vi "LJ Clock.vi"(10 "Sync to second":bool, 11 "Initialize":bool) -> (3 "Seconds since 1/1/1904 universal time":ext format="%.3f")   [LabVIEW 2021]
panel:
  in  "Previous Tick":u32
  in  "Seconds Offset":ext format="%.3f"
  # "Uses the combined values of \"Get Date/Time In Seconds\" and\n\"Tick Count (ms)\" to determine the absolute time (with milliseconds)\nsince midnight on January 1, 1904.\n\nSet \"Initialize\" to TRUE the first time this VI is called.\n\nsupport@labjack.com\nwww.labjack.com"
  # "If the current tick is less\nthan the previous tick, the\nmillisecond timer has rolled."
  # "Offset that must be\nadded to the millisecond\ntimer to get absolute time."
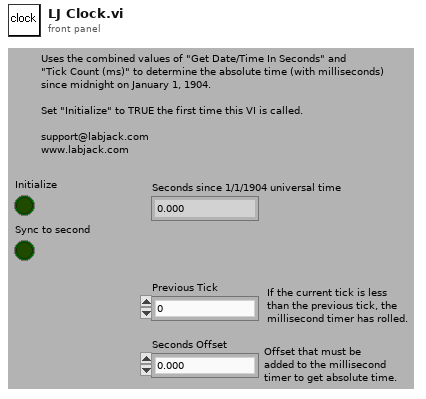
[diagram p1: front panel]
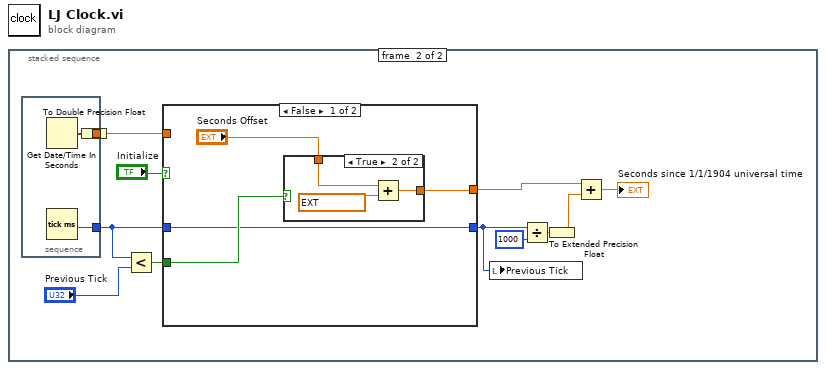
[diagram p0: block diagram]
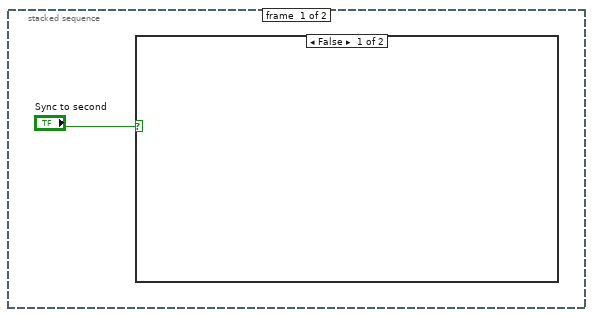
[diagram p2: hidden frame]
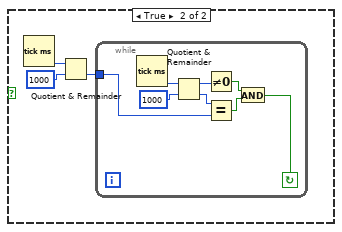
[diagram p3: hidden frame]
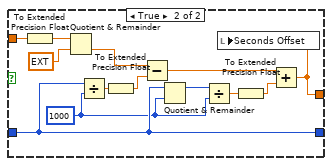
[diagram p5: hidden frame]
diagram:
  n1 = stacked-sequence {
    frame #0 {
      n2 = case shown="False" "Sync to second" {
        frame False {
        }
        frame True {
          n3 = Tick Count (ms)() -> (millisecond timer value=w3:u32)
          n4 = Quotient & Remainder(x=w3, y=u32 1000) -> (floor(x/y)=w2:u32)  [unwired: 1 out]
          n5 = while {
            tunnel: w2 -> [w8]
            stop <- w5 continue-if-true
            n6 = Tick Count (ms)() -> (millisecond timer value=w12:u32)
            n7 = Quotient & Remainder(x=w12, y=u32 1000) -> (x-y*floor(x/y)=w10:u32, floor(x/y)=w9:u32)
            n8 = Not Equal To 0?(x=w10) -> (x != 0?=w7:bool)
            n9 = Equal?(x=w9, y=w8) -> (x = y?=w6:bool)
            n10 = And(x=w7, y=w6) -> (x .and. y?=w5:bool)
          }
        }
      }
    }
    frame #1 {
      n11 = stacked-sequence {
        tunnel: [w26] -> w21
        tunnel: [w25] -> w15
        frame #0 {
          n12 = Get Date/Time In Seconds() -> (seconds since 1Jan1904=w24:timestamp)
          n13 = Tick Count (ms)() -> (millisecond timer value=w26:u32)
          n14 = To Double Precision Float(number=w24) -> (double precision float=w25:dbl)
        }
      }
      n15 = Less?(x=w21, y="Previous Tick") -> (x < y?=w16:bool)
      n16 = case shown="False" "Initialize" {
        tunnel: [w27 w41] -> w17
        tunnel: w21 -> [w28 w46]
        tunnel: [w28 w46] -> w13
        tunnel: w16 -> [w29 _]
        tunnel: w15 -> [_ w38]
        frame False {
          n17 = case shown="True" w29 {
            tunnel: "Seconds Offset" -> [w31 w34]
            tunnel: [w31 w32] -> w27
            frame False {
            }
            frame True {
              n18 = Add(x=w34, y=ext 4294967.2959999999998) -> (x+y=w32:ext)
            }
          }
        }
        frame True {
          w44 = u32 1000 ("y")
          n19 = To Extended Precision Float(1:w38) -> (0:w37:ext)
          n20 = Quotient & Remainder(x=w37, y=ext 1.0) -> (floor(x/y)=w35:ext)  [unwired: 1 out]
          n21 = Divide(x=w46, y=w44) -> (x/y=w47:dbl)
          n22 = To Extended Precision Float(1:w47) -> (0:w40:ext)
          n23 = Subtract(x=w35, y=w40) -> (x-y=w39:ext)
          n24 = Quotient & Remainder(x=w46, y=w44) -> (x-y*floor(x/y)=w45:u32)  [unwired: 1 out]
          n25 = Divide(x=w45, y=w44) -> (x/y=w43:dbl)
          n26 = To Extended Precision Float(1:w43) -> (0:w42:ext)
          n27 = Add(x=w39, y=w42) -> (x+y=w41:ext)
          n28 = local write "Seconds Offset"(w41) -> ()
        }
      }
      n29 = local write "Previous Tick"(w13) -> ()
      n30 = Divide(x=w13, y=u32 1000) -> (x/y=w20:dbl)
      n31 = To Extended Precision Float(1:w20) -> (0:w18:ext)
      n32 = Add(x=w17, y=w18) -> (x+y=→"Seconds since 1/1/1904 universal time":ext)
    }
  }
